vi "Exemple_Extraction_TfidfVectorizer.vi"() -> ()   [LabVIEW 2020]
uses:
  Objet/6 - Datasets Transformation/6.2 - Feature extraction/TfidfVectorizer/TfidfVectorizer.lvclass
panel:
  in  "doc":string
  in  "raw_documents":string[][](array[string])=[["This is the first document."], ["This document is the second document."], ["And this is the third one."], ["Is this the first document?"]]
  in  "TfidfVectorizer":T1={"encoding"="utf-8", "decode_error"="strict", "strip_accents"="None", "lowercase"=TRUE, "preprocessor"="None", "tokenizer"="None", "analyzer"="word", "stop_words"={"Type"="None", "list"=[]}, "token_pattern"="(?u)\\b\\w\\w+\\b", "ngram_range"={"min_n"=1, "max_n"=1}, "max_df"=1.0, "min_df"=1.0, "max_features"=-1, "vocabulary"={"Clé"=["None"], "Valeur"=[]}, "binary"=FALSE, "dtype"="float", "norm"="l2", "use_idf"=TRUE, "smooth_idf"=TRUE, "sublinear_tf"=FALSE} {"max_features" min=-1; "min_df" min=0.0 max=1.0; "max_df" min=0.0 max=1.0}
  out "Data":T2
  out "error out":errorcluster caption="sortie d'erreur"
  in  "error in":errorcluster caption="entrée d'erreur"
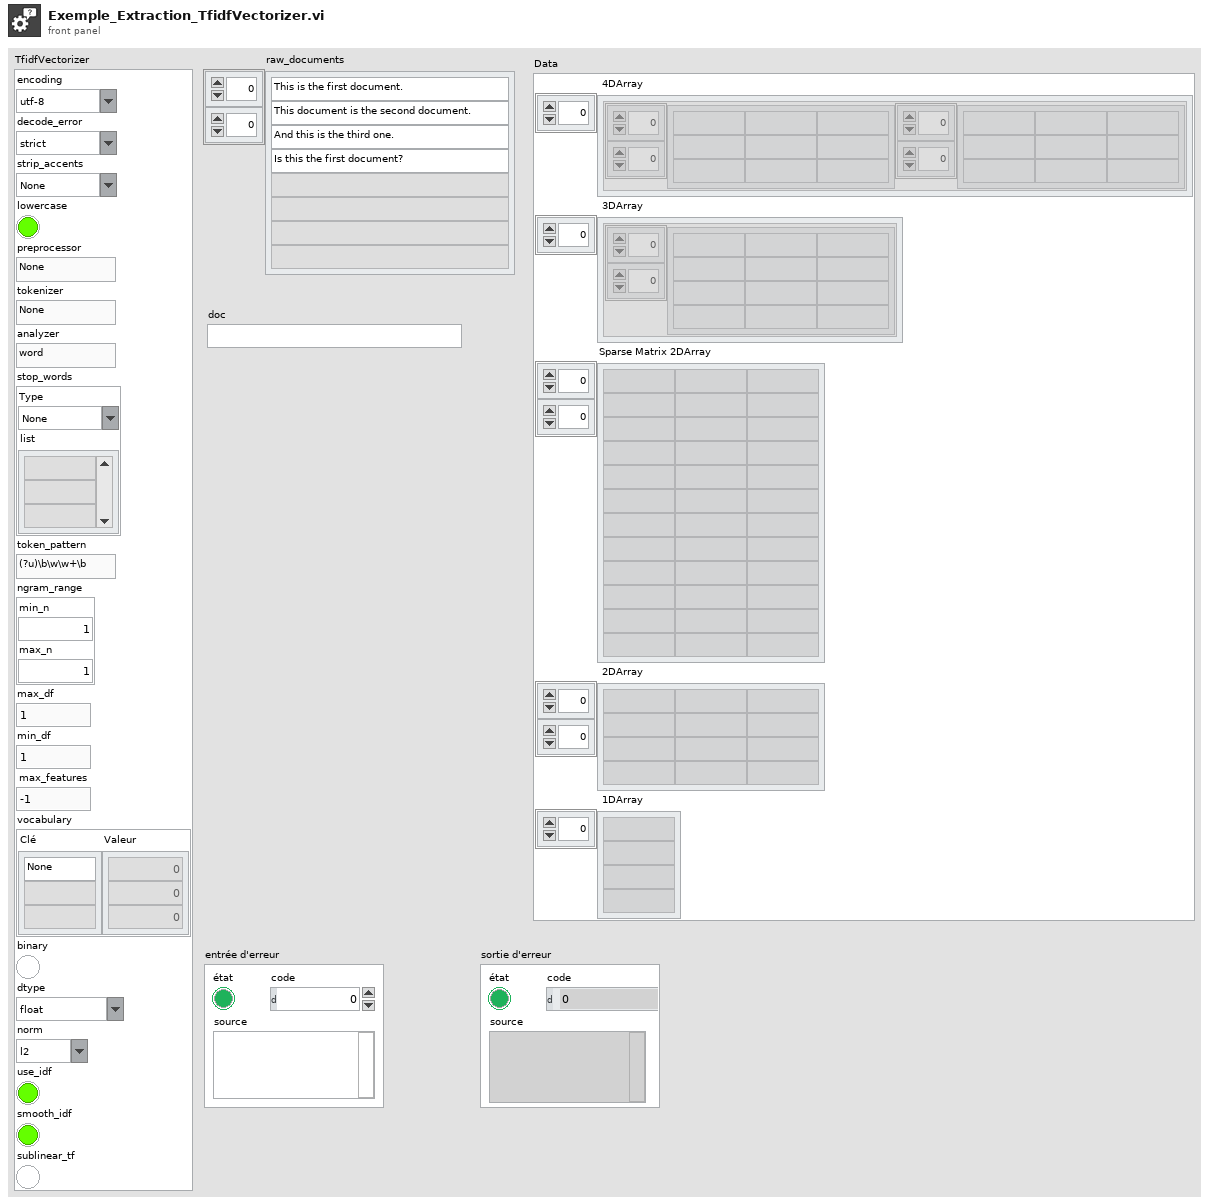
[diagram p1: front panel]
types:
  T1 = cluster{"encoding":string, "decode_error":string, "strip_accents":string, "lowercase":bool, "preprocessor":string, "tokenizer":string, "analyzer":string, "stop_words":cluster{"Type":string, "list":string[]}, "token_pattern":string, "ngram_range":cluster{"min_n":i32, "max_n":i32}, "max_df":dbl, "min_df":dbl, "max_features":i32, "vocabulary":cluster{"Clé":string[], "Valeur":i32[]}, "binary":bool, "dtype":string, "norm":string, "use_idf":bool, "smooth_idf":bool, "sublinear_tf":bool}
  T2 = cluster{" 4DArray":cluster{"1":string[][], "2":string[][]}[], " 3DArray":cluster{"Tableau":string[][]}[], "Sparse Matrix 2DArray":string[][], " 2DArray":string[][], " 1DArray":string[]}
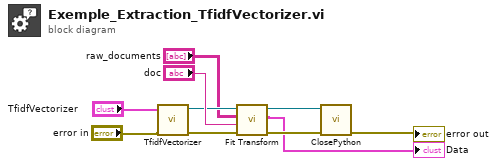
[diagram p0: block diagram]
diagram:
  n1 = call "TfidfVectorizer.vi"("error in"="error in", "TfidfVectorizer"="TfidfVectorizer") -> ("error out"=w7:errorcluster, "TfidfVectorizer.lvclass"=w8:refnum<class "TfidfVectorizer.lvclass">)  [unwired: 8 in]
  n2 = call-dynamic "Fit Transform.vi"("error in (no error)"=w7, "doc"="doc", "X"="raw_documents", "TfidfVectorizer.lvclass"=w8) -> ("error out"=w5:errorcluster, "Data"=→"Data":T2, "TfidfVectorizer.lvclass"=w6:refnum<class "TfidfVectorizer.lvclass">)  [unwired: 5 in]
  n3 = call-dynamic "ClosePython.vi"("error in (no error)"=w5, "Scikit-learn en entrée"=w6) -> ("error out"=→"error out":errorcluster)  [unwired: 8 in, 1 out]
